vi "Read HE ZYState.vi"(8 "error in (no error)":errorcluster, 9 "node IDs":T3=["ns=2;s=GM4TB1.state"], 10 "OPC UA client refnum in":T2, 11 "ZY_State in":T1) -> (0 "error out":errorcluster, 2 "connect":bool, 3 "ZY_State out":T1)   [LabVIEW 2019, in "OPC addons.lvlib"]
uses:
  OPC addons.lvlib
  Heating/ctl/ZY_state_OPC.ctl
  <vilib>/OPCUA/controls/NodeIds.ctl
  <vilib>/OPCUA/controls/NodeId.ctl
  <vilib>/OPCUA/controls/OPC UA Client Refnum.ctl
  79fa441b-c8cd-4727-beae-e2fe135304de.vi
  <vilib>/OPCUA/client/Multiple Read String.vi
  <vilib>/JDP Science/JSONtext/JSON text to Variant.vi
  <vilib>/JDP Science/JSONtext/LVClass Serializer/JSONtext LVClass Serializer.lvclass
  Heating/Heating.lvlib
  <vilib>/OPCUA/NI OPC UA Client.lvlib
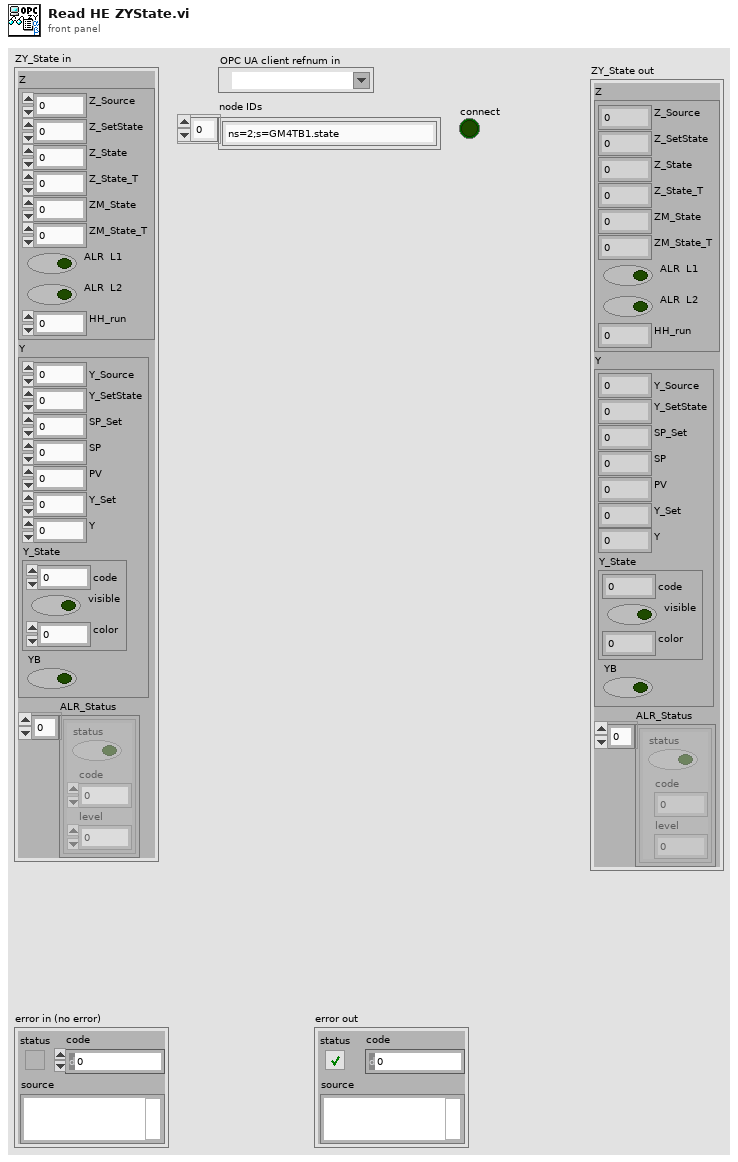
[diagram p1: front panel]
types:
  T1 = typedef "Heating.lvlib/ZY_state_OPC.ctl" = cluster{"Z":cluster{"Z_Source":u8, "Z_SetState":u8, "Z_State":u8, "Z_State_T":u32, "ZM_State":u8, "ZM_State_T":u32, "ALR  L1":bool, "ALR  L2":bool, "HH_run":i32}, "Y":cluster{"Y_Source":u8, "Y_SetState":u8, "SP_Set":dbl, "SP":dbl, "PV":dbl, "Y_Set":dbl, "Y":dbl, "Y_State":cluster{"code":i32, "visible":bool, "color":u32}, "YB":bool}, "ALR_Status":cluster{"status":bool, "code":i32, "level":i32}[]}
  T2 = typedef "OPC UA Client Refnum.ctl" = refnum<k21>
  T3 = typedef "NodeIds.ctl" = T4[]
  T4 = typedef "NodeId.ctl" = string
  T5 = typedef "OPC UA StatusCode.ctl" = u32
  T6 = cluster{"node ID":T4, "value ":string, "timestamp":timestamp, "status":T5}[]
  T7 = cluster{"node ID":T4, "value ":string, "timestamp":timestamp, "status":T5}
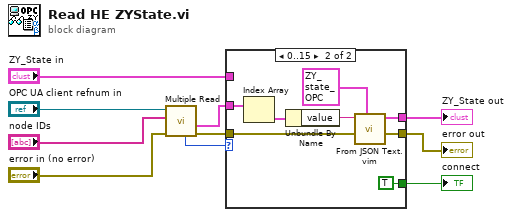
[diagram p0: block diagram]
diagram:
  n1 = call-poly <vilib>:"Multiple Read.vi"("error in (no error)"="error in (no error)", "node IDs"="node IDs", "OPC UA client refnum in"="OPC UA client refnum in") -> ("error out"=w9:errorcluster, "results"=w8:T6, "service status"=w10:T5)  [unwired: 5 in, 1 out]
  n2 = case shown="0..15" w10 {
    tunnel: w9 -> [w12 w18]
    tunnel: [w12 w17] -> w3
    tunnel: w8 -> [_ w16]
    tunnel: [w11 w15] -> w2
    tunnel: [_ TRUE] -> w1
    tunnel: "ZY_State in" -> [w11 _]
    frame 16.., Default {
    }
    frame 0..15 {
      n3 = Index Array(array=w16) -> (element=w20:T7)  [unwired: 1 in]
      n4 = Unbundle By Name(w20) -> ("value"=w19:string)
      n5 = call "From JSON Text.vim"("Data Type and Default Value"=T1 {"Z"={"Z_Source"=0, "Z_SetState"=0, "Z_State"=0, "Z_State_T"=0, "ZM_State"=0, "ZM_State_T"=0, "ALR  L1"=FALSE, "ALR  L2"=FALSE, "HH_run"=0}, "Y"={"Y_Source"=0, "Y_SetState"=0, "SP_Set"=0.0, "SP"=0.0, "PV"=0.0, "Y_Set"=0.0, "Y"=0.0, "Y_State"={"code"=0, "visible"=FALSE, "color"=0}, "YB"=FALSE}, "ALR_Status"=[]} ("ZY_State"), "error in (no error)"=w18, "JSON"=w19) -> ("error out"=w17:errorcluster, "Data out"=w15:T1)  [unwired: 7 in]
    }
  }
  "error out" <- w3
  "ZY_State out" <- w2
  "connect" <- w1
